vi "CENTER STIGMATOR.vi"(0 "STIGMATOR":T2 {"STIG ALIGN"."-Y" min=-100 max=100 step=0.1 scale=-100.0..100.0; "STIG ALIGN"."+Y" min=-100 max=100 step=0.1 scale=-100.0..100.0; "STIG ALIGN"."-X" min=-100 max=100 step=0.1 scale=-100.0..100.0; "STIG ALIGN"."+X" min=-100 max=100 step=0.1 scale=-100.0..100.0; "THETA" format="%_3g"; "OFFY" format="%_3g"; "OFFX" format="%_3g"; "STIG Y" format="%_3g"; "STIG X" format="%_3g"}, 1 "X or Y WOBBLING":bool, 2 "ZOOM":sgl format="%.2f") -> (4 "STIGMATOR COMMAND":string)   [LabVIEW 2018]
uses:
  CENTER STIGMATOR.ctl
panel:
  out "OUTPUT":T1 {"8" format="%_3g"; "7" format="%_3g"; "6" format="%_3g"; "5" format="%_3g"; "4" format="%_3g"; "3" format="%_3g"; "2" format="%_3g"; "1" format="%_3g"}
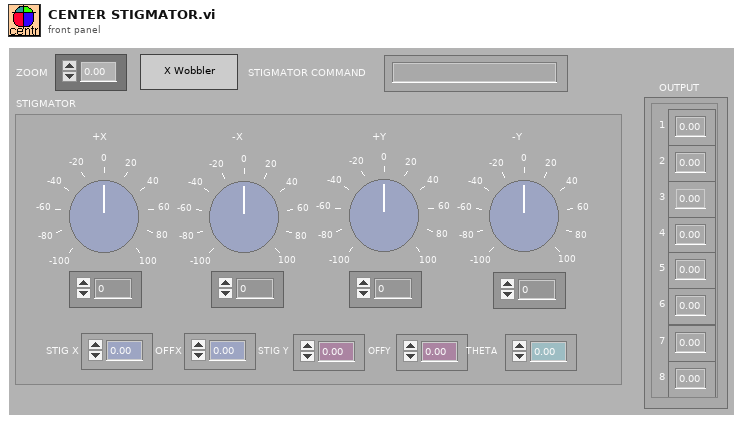
[diagram p1: front panel]
types:
  T1 = cluster{"1":dbl, "output x":dbl, "3":dbl, "4":dbl, "5":dbl, "6":dbl, "7":dbl, "8":dbl}
  T2 = typedef "CENTER STIGMATOR.ctl" = cluster{"STIG ALIGN":cluster{"+X":sgl, "-X":sgl, "+Y":sgl, "-Y":sgl}, "STIG X":dbl, "OFFX":dbl, "STIG Y":dbl, "OFFY":dbl, "THETA":dbl}
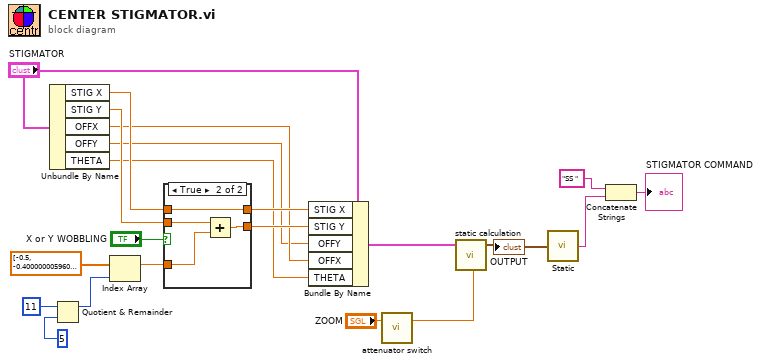
[diagram p0: block diagram]
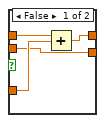
[diagram p2: hidden frame]
diagram:
  n1 = Unbundle By Name("STIGMATOR") -> ("STIG X"=w12:dbl, "STIG Y"=w15:dbl, "OFFX"=w7:dbl, "OFFY"=w6:dbl, "THETA"=w5:dbl)
  n2 = Quotient & Remainder(x=11, y=5) -> (x-y*floor(x/y)=w19:i32)  [unwired: 1 out]
  n3 = Index Array(array=sgl[] [-0.5, -0.4, -0.3, -0.2, -0.1, 0.0, 0.1, 0.2, 0.3, 0.4, 0.5] ("Array"), index=w19) -> (element=w17:sgl)
  n4 = case shown="True" "X or Y WOBBLING" {
    tunnel: [w25 w26] -> w14
    tunnel: w12 -> [w24 w26]
    tunnel: w15 -> [w22 w28]
    tunnel: [w22 w29] -> w13
    tunnel: w17 -> [w23 w27]
    frame False {
      n5 = Add(x=w24, y=w23) -> (x+y=w25:dbl)
    }
    frame True {
      n6 = Add(x=w28, y=w27) -> (x+y=w29:dbl)
    }
  }
  n7 = Bundle By Name(cluster="STIGMATOR", "STIG X"=w14, "STIG Y"=w13, "OFFY"=w6, "OFFX"=w7, "THETA"=w5) -> (w4:T2)
  n8 = call "attenuator switch.vi"("zoom"="ZOOM") -> ("Multiplicateur"=w11:sgl)  [unwired: 1 in, 1 out]
  n9 = call "static calculation.vi"("MULTIPLIER"=w11, "STIGMATOR"=w4) -> ("OUTPUT"=w10:T1)  [unwired: 2 in, 1 out]
  "OUTPUT" <- w10
  n10 = call "Static.vi"("OUTPUT"=w10) -> ("Echo2"=w2:string)  [unwired: 4 in]
  n11 = Concatenate Strings("SS ", w2) -> (→"STIGMATOR COMMAND":string)
